vi "Get Channel Count.vi"(11 "DBL Buffer in":refnum<class "Double Pointer.lvclass">) -> (2 "channel count":u64, 3 "DBL Buffer out":refnum<class "Double Pointer.lvclass">)   [LabVIEW 2017, in "Data Sharing Framework Engine.lvlib" / "Double Pointer.lvclass"]
uses:
  Double Pointer.lvclass
  Double Pointer.lvclass/Double Pointer.ctl
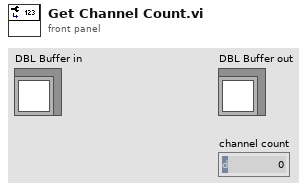
[diagram p1: front panel]
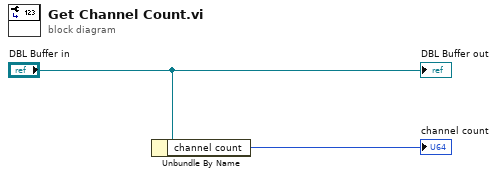
[diagram p0: block diagram]
diagram:
  n1 = Unbundle By Name("DBL Buffer in") -> ("channel count"=→"channel count":u64)
  "DBL Buffer out" <- "DBL Buffer in"
